vi "Write Countdown Length (sec).vi"(8 "error in (no error)":errorcluster, 10 "Countdown Length (sec)":dbl, 11 "Countdown Timer in":refnum<class "Countdown Timer.lvclass">) -> (0 "error out":errorcluster, 3 "Countdown Timer out":refnum<class "Countdown Timer.lvclass">)   [LabVIEW 2015, in "Countdown Timer.lvlib" / "Countdown Timer.lvclass"]
uses:
  Countdown Timer.lvclass
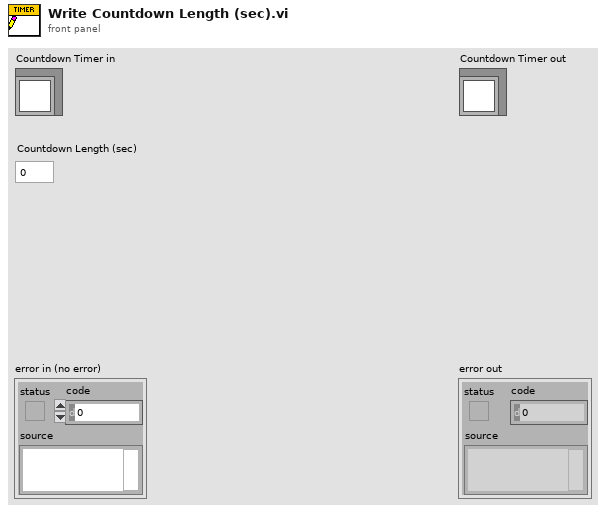
[diagram p1: front panel]
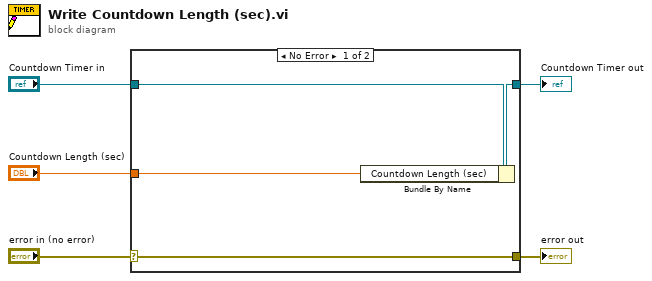
[diagram p0: block diagram]
diagram:
  n1 = case shown="No Error" "error in (no error)" {
    selector: "error in (no error)" -> [w9 w10]
    tunnel: [w9 w10] -> w4
    tunnel: [w7 w11] -> w2
    tunnel: "Countdown Timer in" -> [w8 w11]
    tunnel: "Countdown Length (sec)" -> [w6 _]
    frame No Error {
      n2 = Bundle By Name(cluster=w8, "Countdown Length (sec)"=w6) -> (w7:refnum<class "Countdown Timer.lvclass">)
    }
    frame Error {
    }
  }
  "error out" <- w4
  "Countdown Timer out" <- w2
